vi "Write.Lookup.vi"(8 "error in (no error)":errorcluster, 10 "Name":string, 11 "Data Access API in":refnum<class "Data Access Engine.lvclass">) -> (0 "error out":errorcluster, 2 "Ref":refnum<data-value>, 3 "Data Access API out":refnum<class "Data Access Engine.lvclass">)   [LabVIEW 2015, in "Data Access Engine.lvlib" / "Data Access Engine.lvclass"]
uses:
  Data Access Engine.lvclass
  Access Type Classes/Write/Write.lvclass
  Data Access Engine.lvclass/Data Access Engine.ctl
  Types/VS Channel Group Type.ctl
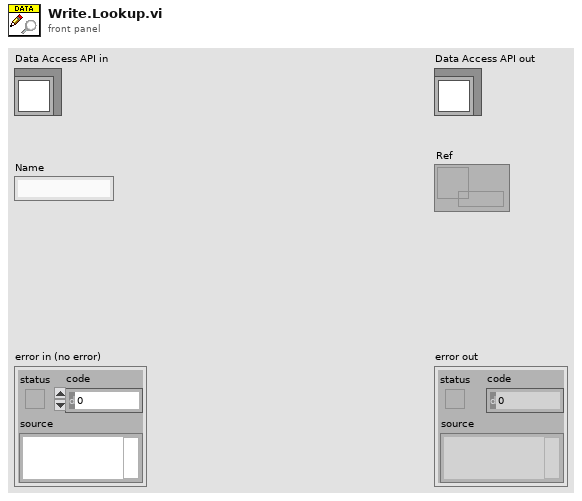
[diagram p1: front panel]
types:
  T1 = typedef "Data Access Engine.lvlib/Data Access Engine.lvclass/VS Channel Group Type.ctl" = enum16{"Output/Write", "Input/Read", "Input/ReadWrite"}
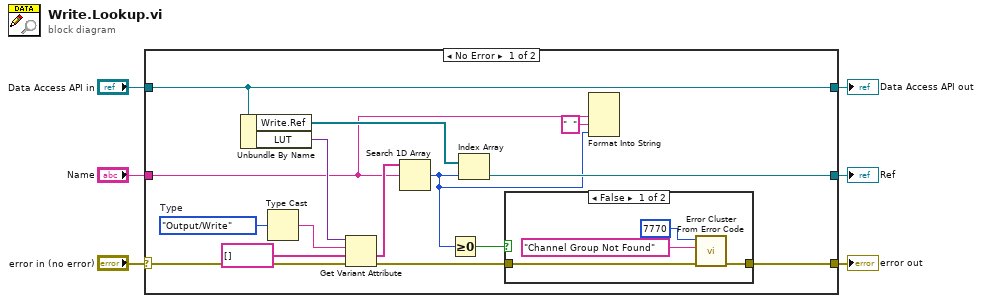
[diagram p0: block diagram]
diagram:
  n1 = case shown="No Error" "error in (no error)" {
    selector: "error in (no error)" -> [w17 w28]
    tunnel: [w10 w28] -> w5
    tunnel: [w21 w27] -> w3
    tunnel: "Data Access API in" -> [w21 w27]
    tunnel: "Name" -> [w7 _]
    tunnel: [w14 _] -> w1
    frame No Error {
      w13 = VS_Channel_Group_Type."Output/Write"  # Type
      n2 = Unbundle By Name(w21) -> ("Write.Ref"=w15:refnum<data-value>[], "LUT"=w20:variant)
      n3 = Type Cast(x=w13) -> (*(type *) &x=w19:string)  [unwired: 1 in]
      n4 = Get Variant Attribute(Variant=w20, name=w19, default value (empty Variant)=string[] [], error in=w17) -> (value=w16:string[], error out=w12:errorcluster)  [unwired: 2 out]
      n5 = Search 1D Array(1D array=w16, element=w7) -> (index of element=w8:i32)  [unwired: 1 in]
      n6 = Greater Or Equal To 0?(x=w8) -> (x >= 0?=w11:bool)
      n7 = Index Array(array=w15, index=w8) -> (element=w14:refnum<data-value>)
      n8 = case shown="False" w11 {
        tunnel: w12 -> [w25 w26]
        tunnel: [w24 w26] -> w10
        frame False {
          n9 = call <vilib>:"Error Cluster From Error Code.vi"("error in (no error)"=w25, "error message (\"\")"="Channel Group Not Found" ("error message (\"\")"), "error code (0)"=7770) -> ("error out"=w24:errorcluster)  [unwired: 6 in]
        }
        frame True {
        }
      }
      n10 = Format Into String(w7, "  " ("input 2"), w8) -> ()  [unwired: 3 in, 2 out]
    }
    frame Error {
    }
  }
  "error out" <- w5
  "Data Access API out" <- w3
  "Ref" <- w1
